vi "subParseSolutionFile.vi"(8 "error in (no error)":errorcluster, 11 "Solution file":path) -> (0 "error out":errorcluster, 1 "Active targets":string[](array[string]), 2 "Lib definition strings":string[](array[string]), 3 "Projects":path[](array[path]), 4 "Version string":string)   [LabVIEW 2019, in "SolutionBuilder.lvlib" / "SolutionBuilder.lvclass"]
uses:
  SolutionBuilder.lvclass
  <vilib>/xml/Load XML File.vi
  <vilib>/xml/Close Reference(Node).vi
  <vilib>/xml/NI_XML.lvlib
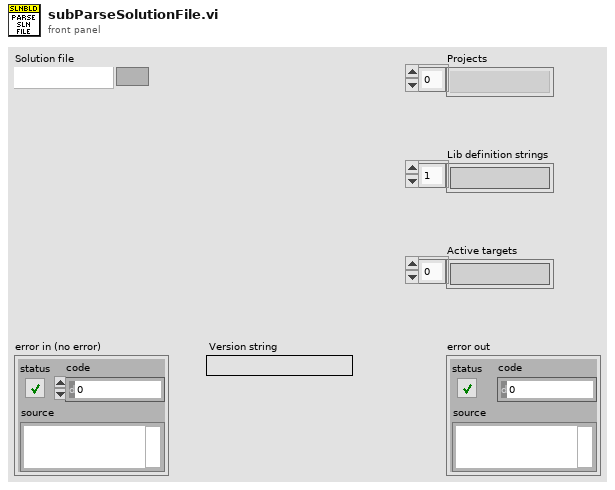
[diagram p1: front panel]
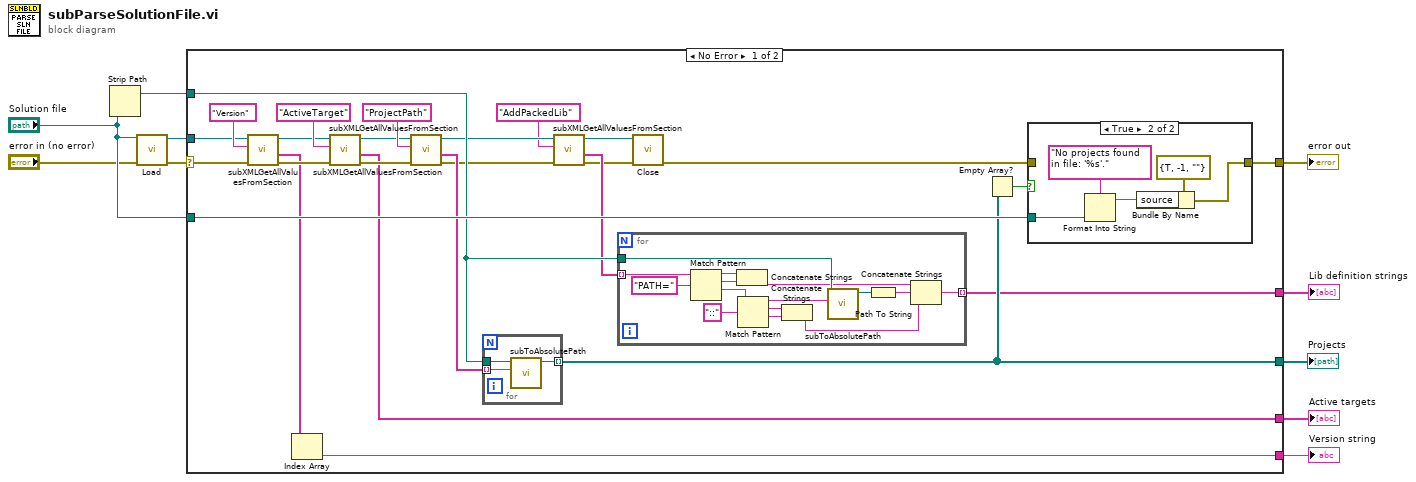
[diagram p0: block diagram]
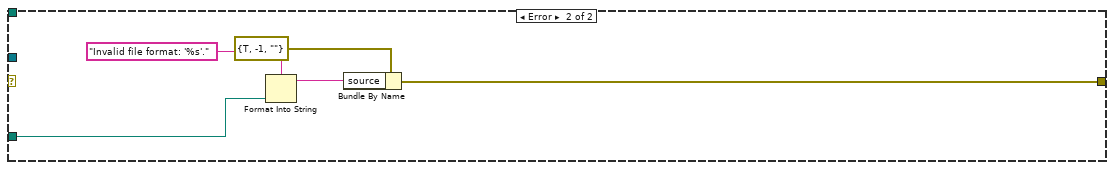
[diagram p3: hidden frame]
diagram:
  n1 = Strip Path(path="Solution file") -> (stripped path=w5:path)  [unwired: 1 out]
  n2 = call-poly <vilib>:"Load.vi"("path to XML document"="Solution file", "error in (no error)"="error in (no error)") -> ("DOM document out"=w4:refnum<k20>, "error out"=w8:errorcluster)  [unwired: 11 in, 1 out]
  n3 = case shown="No Error" w8 {
    selector: w8 -> [w16 _]
    tunnel: w4 -> [w15 _]
    tunnel: w5 -> [w30 _]
    tunnel: [w33 _] -> w6
    tunnel: "Solution file" -> [w34 w61]
    tunnel: [w35 w60] -> w10
    tunnel: [w31 _] -> w3
    tunnel: [w18 _] -> w2
    tunnel: [w11 _] -> w1
    frame No Error {
      n4 = call "subXMLGetAllValuesFromSection.vi"("error in (no error)"=w16, "XPath expression"="Version", "Refnum in"=w15) -> ("error out"=w13:errorcluster, "Values"=w12:string[], "Refnum out"=w14:refnum<k20>)  [unwired: 6 in]
      n5 = Index Array(array=w12) -> (element=w11:string)  [unwired: 1 in]
      n6 = call "subXMLGetAllValuesFromSection.vi"("error in (no error)"=w13, "XPath expression"="ActiveTarget", "Refnum in"=w14) -> ("error out"=w19:errorcluster, "Values"=w18:string[], "Refnum out"=w20:refnum<k20>)  [unwired: 6 in]
      n7 = call "subXMLGetAllValuesFromSection.vi"("error in (no error)"=w19, "XPath expression"="ProjectPath", "Refnum in"=w20) -> ("error out"=w27:errorcluster, "Values"=w28:string[], "Refnum out"=w26:refnum<k20>)  [unwired: 6 in]
      n8 = for {
        tunnel: [w58] -> w33 mode=indexing
        tunnel: w30 -> [w59]
        tunnel: w28 -> [w57] mode=indexing
        n9 = call "subToAbsolutePath.vi"("Path string"=w57, "Root path"=w59) -> ("Path"=w58:path)  [unwired: 9 in]
      }
      n10 = call "subXMLGetAllValuesFromSection.vi"("error in (no error)"=w27, "XPath expression"="AddPackedLib", "Refnum in"=w26) -> ("error out"=w22:errorcluster, "Values"=w24:string[], "Refnum out"=w21:refnum<k20>)  [unwired: 6 in]
      n11 = for {
        tunnel: [w43] -> w31 mode=indexing
        tunnel: w30 -> [w56]
        tunnel: w24 -> [w42] mode=indexing
        n12 = Match Pattern(string=w42, regular expression="PATH=") -> (before substring=w47:string, match substring=w48:string, after substring=w54:string)  [unwired: 1 in, 1 out]
        n13 = Concatenate Strings(w47, w48) -> (w45:string)
        n14 = Match Pattern(string=w54, regular expression="::") -> (before substring=w52:string, match substring=w50:string, after substring=w49:string)  [unwired: 1 in, 1 out]
        n15 = Concatenate Strings(w50, w49) -> (w44:string)
        n16 = call "subToAbsolutePath.vi"("Path string"=w52, "Root path"=w56) -> ("Path"=w51:path)  [unwired: 9 in]
        n17 = Path To String(path=w51) -> (string=w46:string)
        n18 = Concatenate Strings(w45, w46, w44) -> (w43:string)
      }
      n19 = call-poly <vilib>:"Close.vi"("error in (no error)"=w22, "node"=w21) -> ("error out"=w32:errorcluster)  [unwired: 7 in]
      n20 = Empty Array?(array=w33) -> (empty?=w36:bool)
      n21 = case shown="True" w36 {
        tunnel: [_ w38] -> w35
        tunnel: w34 -> [_ w37]
        tunnel: w32 -> [_ _]
        frame False {
        }
        frame True {
          n22 = Format Into String(format string="No projects found in file: '%s'.", w37) -> (resulting string=w40:string)  [unwired: 2 in, 1 out]
          n23 = Bundle By Name(cluster=errorcluster {"status"=TRUE, "code"=-1, "source"=""} ("t"), "source"=w40) -> (w38:errorcluster)
        }
      }
    }
    frame Error {
      n24 = Format Into String(format string="Invalid file format: '%s'.", w61) -> (resulting string=w63:string)  [unwired: 2 in, 1 out]
      n25 = Bundle By Name(cluster=errorcluster {"status"=TRUE, "code"=-1, "source"=""} ("t"), "source"=w63) -> (w60:errorcluster)
    }
  }
  "error out" <- w10
  "Projects" <- w6
  "Lib definition strings" <- w3
  "Active targets" <- w2
  "Version string" <- w1
